vi "2014 Vision Math V 1.vi"(9 "target width (ft)":dbl, 10 "target height (ft)":dbl, 11 "distance(ft)":dbl) -> (1 "theta H":dbl, 2 "theta W":dbl, 3 "H/W to true center":cluster{dbl, dbl})   [LabVIEW 2013]
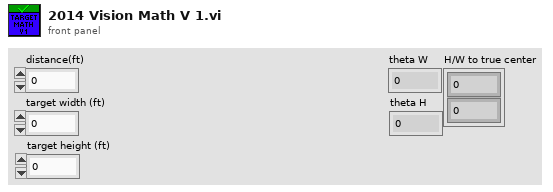
[diagram p1: front panel]
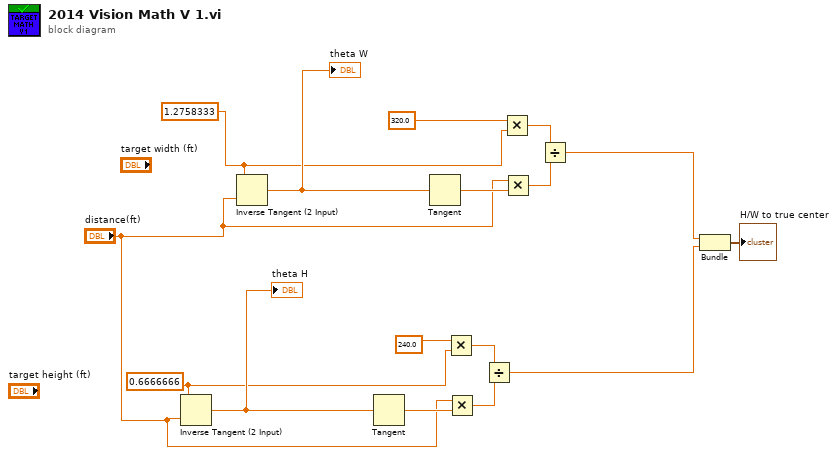
[diagram p0: block diagram]
diagram:
  w1 = 0.6666666 ("x")
  w2 = 1.2758333 ("x")
  n1 = Inverse Tangent (2 Input)(1:"distance(ft)", 2:w1) -> (0:w8:dbl)
  "theta H" <- w8
  n2 = Inverse Tangent (2 Input)(1:"distance(ft)", 2:w2) -> (0:w13:dbl)
  "theta W" <- w13
  n3 = Tangent(1:w8) -> (0:w9:dbl)
  n4 = Tangent(1:w13) -> (0:w14:dbl)
  n5 = Multiply(x=240.0 ("FOV pixels H"), y=w1) -> (x*y=w11:dbl)
  n6 = Multiply(x="distance(ft)", y=w9) -> (x*y=w10:dbl)
  n7 = Divide(x=w11, y=w10) -> (x/y=w5:dbl)
  n8 = Multiply(x=320.0 ("FOV pixels W"), y=w2) -> (x*y=w16:dbl)
  n9 = Multiply(x="distance(ft)", y=w14) -> (x*y=w15:dbl)
  n10 = Divide(x=w16, y=w15) -> (x/y=w6:dbl)
  n11 = Bundle(w6, w5) -> (→"H/W to true center":cluster{dbl, dbl})  [unwired: 1 in]
